vi "AMZ_S3_APIHLP_Parse Set Bucket Website Request Parameters.vi"(8 "error in (no error)":errorcluster, 11 "Website Configuration":T1) -> (0 "error out":errorcluster, 5 "PUT Data":string)   [LabVIEW 2015, in "LV Interface for Amazon S3.lvlib"]
uses:
  LV Interface for Amazon S3.lvlib
  Typedefs/AMZ_S3_API_WebsiteConfiguration.ctl
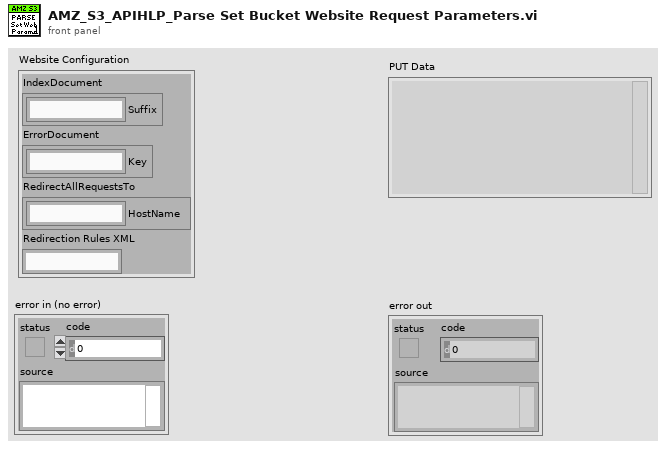
[diagram p1: front panel]
types:
  T1 = typedef "LV Interface for Amazon S3.lvlib/AMZ_S3_API_WebsiteConfiguration.ctl" = cluster{"IndexDocument":cluster{"Suffix":string}, "ErrorDocument":cluster{"Key":string}, "RedirectAllRequestsTo":cluster{"HostName":string}, "Redirection Rules XML":string}
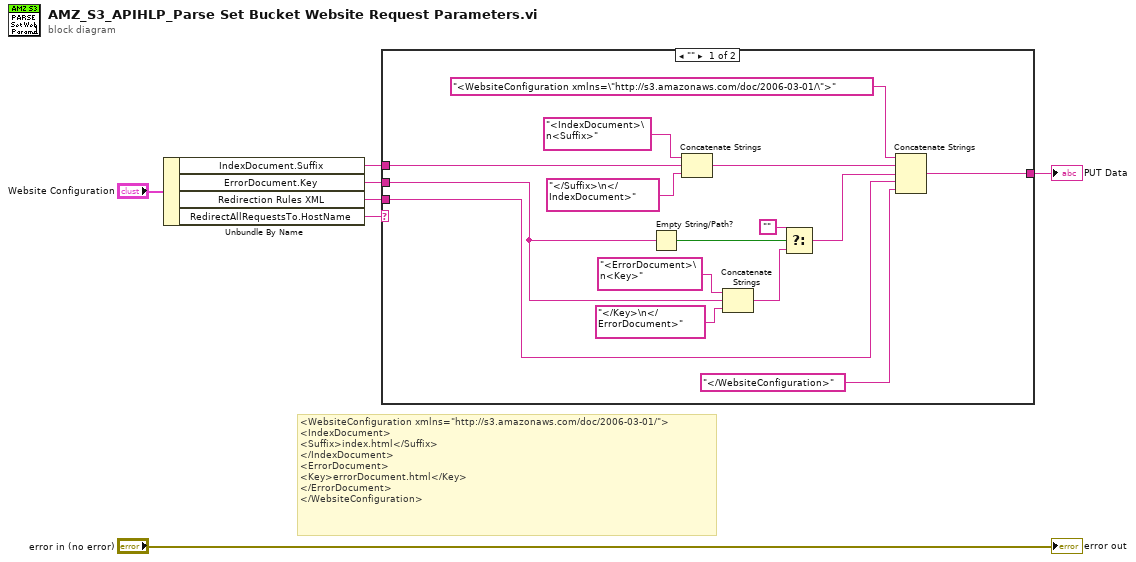
[diagram p0: block diagram]
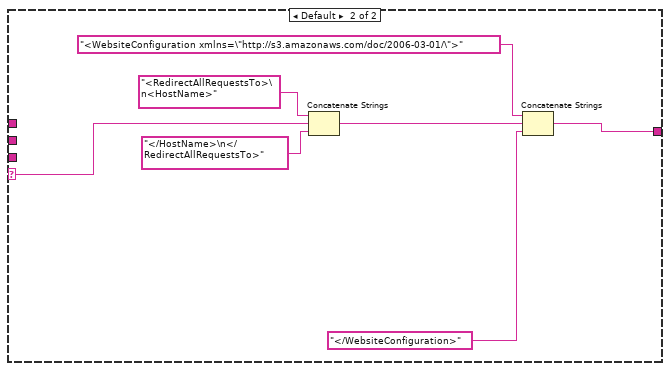
[diagram p2: hidden frame]
diagram:
  # "<WebsiteConfiguration xmlns=\"http://s3.amazonaws.com/doc/2006-03-01/\">\n<IndexDocument>\n<Suffix>index.html</Suffix>\n</IndexDocument>\n<ErrorDocument>\n<Key>errorDocument.html</Key>\n</ErrorDocument>\n</WebsiteConfiguration>"
  n1 = Unbundle By Name("Website Configuration") -> ("IndexDocument.Suffix"=w7:string, "ErrorDocument.Key"=w3:string, "Redirection Rules XML"=w1:string, "RedirectAllRequestsTo.HostName"=w2:string)
  n2 = case shown="\"\"" w2 {
    selector: w2 -> [_ w23]
    tunnel: w7 -> [w21 _]
    tunnel: [w11 w25] -> w4
    tunnel: w3 -> [w10 _]
    tunnel: w1 -> [w8 _]
    frame "" {
      n3 = Empty String/Path?(string/path=w10) -> (empty?=w17:bool)
      n4 = Concatenate Strings("<IndexDocument>\n<Suffix>", w21, "</Suffix>\n</IndexDocument>") -> (w13:string)
      n5 = Concatenate Strings("<ErrorDocument>\n<Key>", w10, "</Key>\n</ErrorDocument>") -> (w16:string)
      n6 = Select(t="", s=w17, f=w16) -> (s? t:f=w12:string)
      n7 = Concatenate Strings("<WebsiteConfiguration xmlns=\"http://s3.amazonaws.com/doc/2006-03-01/\">", w13, w12, w8, "</WebsiteConfiguration>") -> (w11:string)
    }
    frame Default {
      n8 = Concatenate Strings("<RedirectAllRequestsTo>\n<HostName>", w23, "</HostName>\n</RedirectAllRequestsTo>") -> (w26:string)
      n9 = Concatenate Strings("<WebsiteConfiguration xmlns=\"http://s3.amazonaws.com/doc/2006-03-01/\">", w26, "</WebsiteConfiguration>") -> (w25:string)
    }
  }
  "PUT Data" <- w4
  "error out" <- "error in (no error)"
